vi "MotorManager_3614.vi"(3 "error in (no error)":errorcluster caption="错误输入（无错误）", 4 "Input":T2, 5 "ref_in":T1) -> (0 "error out":errorcluster caption="错误输出", 1 "Output":T2, 2 "ref_out":T1)   [LabVIEW 2012]
uses:
  D:/github/LVsolis/AGUC2/AgilisCmdLib.dll
  AGUC2/AgilisCmdLib.dll
  D:/github/LVsolis/lib/CmdLib.dll
  lib/CmdLib.dll
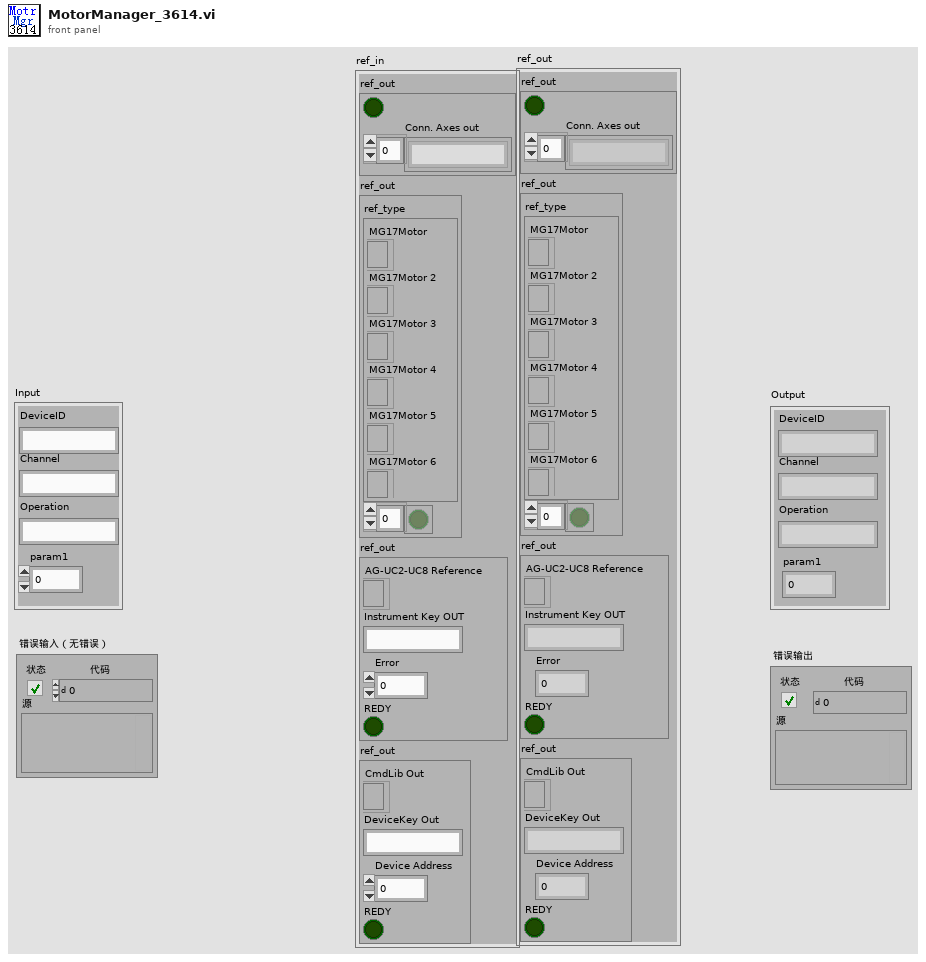
[diagram p1: front panel]
types:
  T1 = cluster{"ref_out":cluster{bool, "Conn. Axes out":string[]}, "ref_out":cluster{"ref_type":cluster{"MG17Motor":refnum<k7>, "MG17Motor 2":refnum<k7>, "MG17Motor 3":refnum<k7>, "MG17Motor 4":refnum<k7>, "MG17Motor 5":refnum<k7>, "MG17Motor 6":refnum<k7>}, bool[]}, "ref_out":cluster{"AG-UC2-UC8 Reference":refnum<k24>, "Instrument Key OUT":string, "Error":i32, "REDY":bool}, "ref_out":cluster{"CmdLib Out":refnum<k24>, "DeviceKey Out":string, "Device Address":i32, "REDY":bool}}
  T2 = cluster{"DeviceID":string, "Channel":string, "param1":dbl, "Operation":string}
  T3 = cluster{"ref_type":cluster{"MG17Motor":refnum<k7>, "MG17Motor 2":refnum<k7>, "MG17Motor 3":refnum<k7>, "MG17Motor 4":refnum<k7>, "MG17Motor 5":refnum<k7>, "MG17Motor 6":refnum<k7>}, bool[]}
  T4 = cluster{"AG-UC2-UC8 Reference":refnum<k24>, "Instrument Key OUT":string, "Error":i32, "REDY":bool}
  T5 = cluster{"CmdLib Out":refnum<k24>, "DeviceKey Out":string, "Device Address":i32, "REDY":bool}
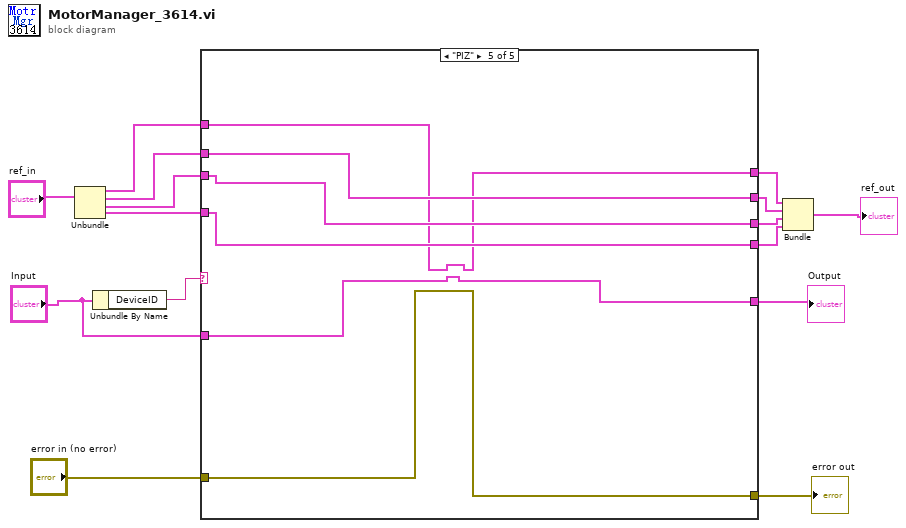
[diagram p0: block diagram]
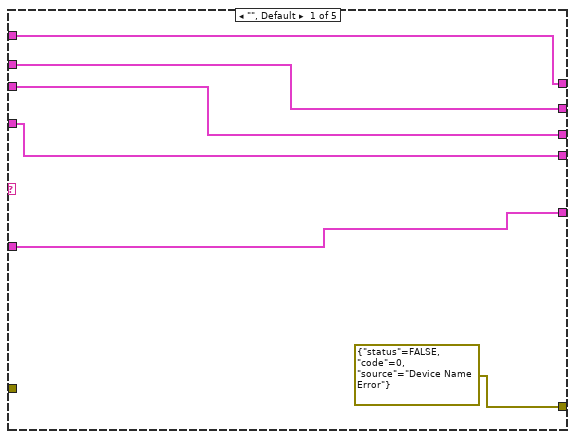
[diagram p2: hidden frame]
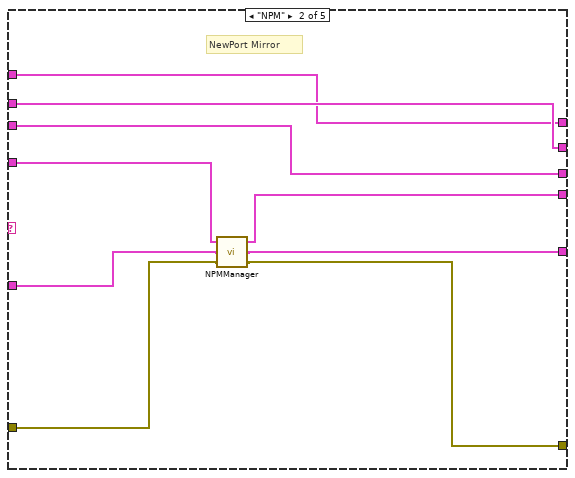
[diagram p3: hidden frame]
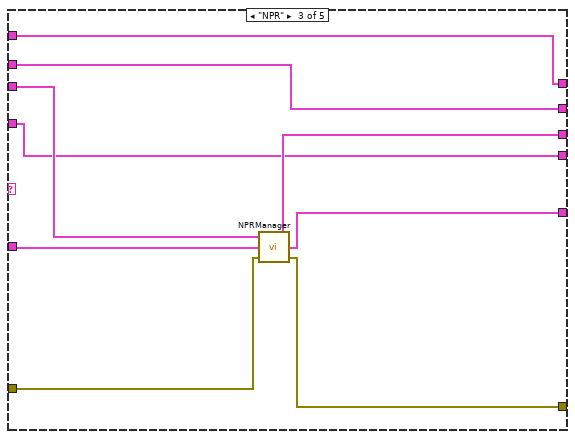
[diagram p4: hidden frame]
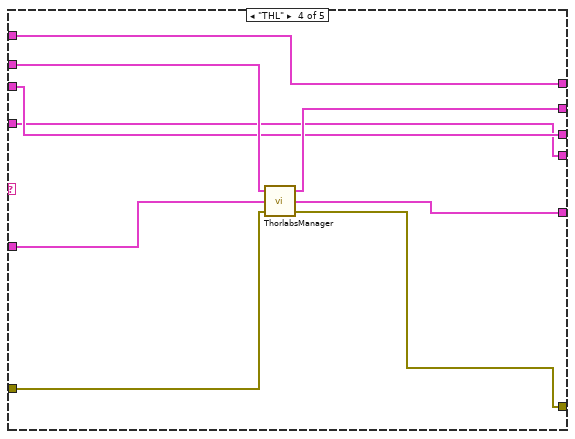
[diagram p5: hidden frame]
diagram:
  n1 = Unbundle("ref_in") -> ("ref_out"=w5:cluster{bool, "Conn. Axes out":string[]}, "ref_out"=w2:T3, "ref_out"=w3:T4, "ref_out"=w4:T5)
  n2 = Unbundle By Name("Input") -> ("DeviceID"=w15:string)
  n3 = case shown="\"PIZ\"" w15 {
    tunnel: "Input" -> [w21 w27 w37 w46 w51]
    tunnel: [w21 w28 w36 w45 w51] -> w13
    tunnel: "error in (no error)" -> [_ w30 w39 w47 w49]
    tunnel: [errorcluster {"status"=FALSE, "code"=0, "source"="Device Name Error"} ("error out") w29 w38 w48 w49] -> w11
    tunnel: [w19 w26 w33 w41 w52] -> w9
    tunnel: [w18 w24 w35 w42 w53] -> w10
    tunnel: w3 -> [w18 w24 w34 w42 w53]
    tunnel: w4 -> [w19 w25 w33 w41 w52]
    tunnel: [w17 w23 w32 w44 w54] -> w8
    tunnel: w2 -> [w17 w23 w32 w43 w54]
    tunnel: [w16 w22 w31 w40 w50] -> w7
    tunnel: w5 -> [w16 w22 w31 w40 w50]
    frame "", Default {
    }
    frame "NPM" {
      # "NewPort Mirror"
      n4 = call "NPMManager.vi"("error in (no error)"=w30, "Input"=w27, "ref_in"=w25) -> ("error out"=w29:errorcluster, "Output"=w28:T2, "ref_out"=w26:T5)
    }
    frame "NPR" {
      n5 = call "NPRManager.vi"("error in (no error)"=w39, "Input"=w37, "ref_in"=w34) -> ("error out"=w38:errorcluster, "Output"=w36:T2, "ref_out"=w35:T4)
    }
    frame "THL" {
      n6 = call "ThorlabsManager.vi"("error in (no error)"=w47, "Input"=w46, "ref_in"=w43) -> ("error out"=w48:errorcluster, "Output"=w45:T2, "ref_out"=w44:T3)
    }
    frame "PIZ" {
    }
  }
  "error out" <- w11
  "Output" <- w13
  n7 = Bundle("ref_out"=w7, "ref_out"=w8, "ref_out"=w10, "ref_out"=w9) -> (→"ref_out":T1)  [unwired: 1 in]
